vi "Set Pump Parameters (SubVI).vi"(0 "Units":string, 1 "error in":errorcluster, 2 "Target Volume":dbl, 5 "Flow rate":dbl, 6 "Direction":string(combo), 7 "Pump Add":string, 8 "diameter (mm)":dbl, 9 "Send":bool, 10 "VISA resource name in":refnum<visa-resource-name>) -> (3 "VISA resource name out":refnum<visa-resource-name>, 4 "error out":errorcluster)   [LabVIEW 2020]
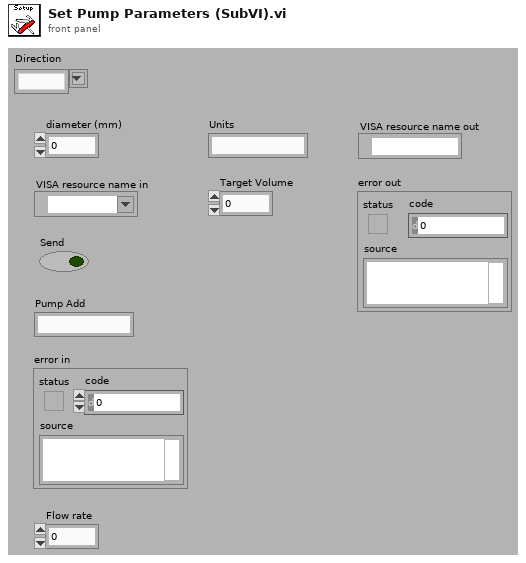
[diagram p1: front panel]
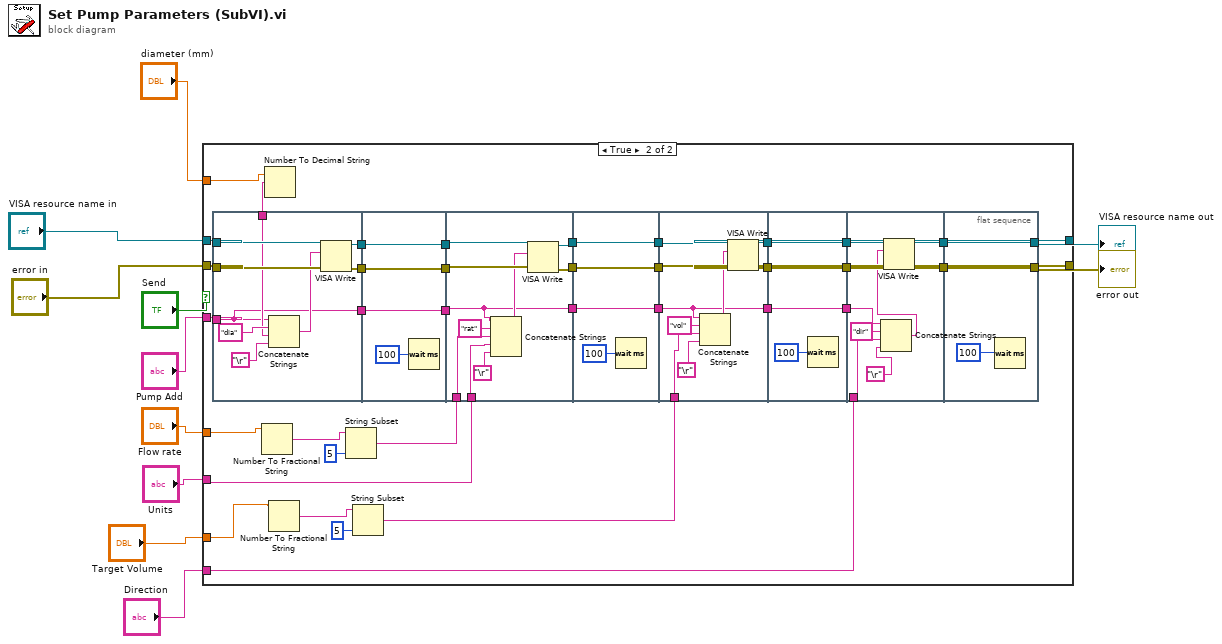
[diagram p0: block diagram]
diagram:
  n1 = case shown="True" "Send" {
    tunnel: "VISA resource name in" -> [w13 w50]
    tunnel: "error in" -> [w12 w49]
    tunnel: [w13 w48] -> w10
    tunnel: [w12 w47] -> w11
    tunnel: "Pump Add" -> [_ w46]
    tunnel: "diameter (mm)" -> [_ w45]
    tunnel: "Flow rate" -> [_ w21]
    tunnel: "Units" -> [_ w43]
    tunnel: "Target Volume" -> [_ w15]
    tunnel: "Direction" -> [_ w24]
    frame False {
    }
    frame True {
      n2 = flat-sequence {
        tunnel: w50 -> [w59]
        tunnel: w49 -> [w58]
        tunnel: [w57] -> w42
        tunnel: [w56] -> w40
        tunnel: w46 -> [w51]
        tunnel: w44 -> [w54]
        tunnel: [w51] -> w38
        tunnel: w42 -> [w63]
        tunnel: [w63] -> w41
        tunnel: w40 -> [w62]
        tunnel: [w62] -> w39
        tunnel: w38 -> [w61]
        tunnel: [w61] -> w37
        tunnel: w41 -> [w73]
        tunnel: w39 -> [w71]
        tunnel: w37 -> [w64]
        tunnel: w19 -> [w68]
        tunnel: w43 -> [w67]
        tunnel: [w72] -> w36
        tunnel: [w70] -> w34
        tunnel: [w64] -> w32
        tunnel: w36 -> [w77]
        tunnel: [w77] -> w35
        tunnel: w34 -> [w76]
        tunnel: [w76] -> w33
        tunnel: w32 -> [w75]
        tunnel: [w75] -> w31
        tunnel: w35 -> [w84]
        tunnel: w33 -> [w83]
        tunnel: w31 -> [w78]
        tunnel: w14 -> [w80]
        tunnel: [w85] -> w30
        tunnel: [w86] -> w29
        tunnel: [w78] -> w26
        tunnel: w30 -> [w90]
        tunnel: w29 -> [w89]
        tunnel: [w90] -> w28
        tunnel: [w89] -> w27
        tunnel: w26 -> [w87]
        tunnel: [w87] -> w25
        tunnel: w28 -> [w99]
        tunnel: w27 -> [w96]
        tunnel: w25 -> [w93]
        tunnel: w24 -> [w91]
        tunnel: [w98] -> w23
        tunnel: [w97] -> w22
        tunnel: [w101] -> w47
        tunnel: [w102] -> w48
        tunnel: w23 -> [w102]
        tunnel: w22 -> [w101]
        frame #0 {
          n3 = Concatenate Strings(w51, "dia" ("string"), w54, "\r") -> (w53:string)
          n4 = VISA Write(VISA resource name=w59, write buffer=w53, error in (no error)=w58) -> (VISA resource name out=w57:refnum<visa-resource-name>, error out=w56:errorcluster)  [unwired: 1 out]
        }
        frame #1 {
          n5 = Wait (ms)(milliseconds to wait=u32 100) -> ()  [unwired: 1 out]
        }
        frame #2 {
          n6 = Concatenate Strings(w64, "rat" ("string"), w68, w67, "\r") -> (w65:string)
          n7 = VISA Write(VISA resource name=w73, write buffer=w65, error in (no error)=w71) -> (VISA resource name out=w72:refnum<visa-resource-name>, error out=w70:errorcluster)  [unwired: 1 out]
        }
        frame #3 {
          n8 = Wait (ms)(milliseconds to wait=u32 100) -> ()  [unwired: 1 out]
        }
        frame #4 {
          n9 = Concatenate Strings(w78, "vol" ("string"), w80, "\r") -> (w79:string)
          n10 = VISA Write(VISA resource name=w84, write buffer=w79, error in (no error)=w83) -> (VISA resource name out=w85:refnum<visa-resource-name>, error out=w86:errorcluster)  [unwired: 1 out]
        }
        frame #5 {
          n11 = Wait (ms)(milliseconds to wait=u32 100) -> ()  [unwired: 1 out]
        }
        frame #6 {
          n12 = Concatenate Strings(w93, "dir" ("string"), w91, "\r") -> (w95:string)
          n13 = VISA Write(VISA resource name=w99, write buffer=w95, error in (no error)=w96) -> (VISA resource name out=w98:refnum<visa-resource-name>, error out=w97:errorcluster)  [unwired: 1 out]
        }
        frame #7 {
          n14 = Wait (ms)(milliseconds to wait=u32 100) -> ()  [unwired: 1 out]
        }
      }
      n15 = Number To Fractional String(number=w21) -> (F-format string=w18:string)  [unwired: 3 in]
      n16 = Number To Decimal String(number=w45) -> (decimal integer string=w44:string)  [unwired: 1 in]
      n17 = Number To Fractional String(number=w15) -> (F-format string=w17:string)  [unwired: 3 in]
      n18 = String Subset(string=w18, length (rest)=5 ("length (rest)")) -> (substring=w19:string)  [unwired: 1 in]
      n19 = String Subset(string=w17, length (rest)=5 ("length (rest)")) -> (substring=w14:string)  [unwired: 1 in]
    }
  }
  "error out" <- w11
  "VISA resource name out" <- w10
